vi "Newport ITX-D3N Range Check.vi"(4 "All Out of Range?":bool, 6 "In Range?":bool, 7 "Barometric Pressure":dbl, 8 "Error In":errorcluster, 9 "Humidity":dbl, 10 "Temperature":dbl, 11 "Dewpoint":dbl) -> (0 "Error Out":errorcluster, 1 "Humidity Out":dbl, 2 "Temperature Out":dbl, 3 "Dewpoint Out":dbl, 5 "Barometric Pressure Out":dbl)   [LabVIEW 2020]
uses:
  <vilib>/Analysis/baseanly.llb/Mean (DBL).vi
  <vilib>/Analysis/NI_AALBase.lvlib
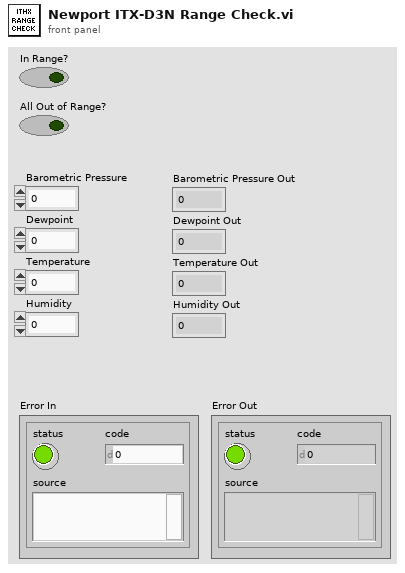
[diagram p1: front panel]
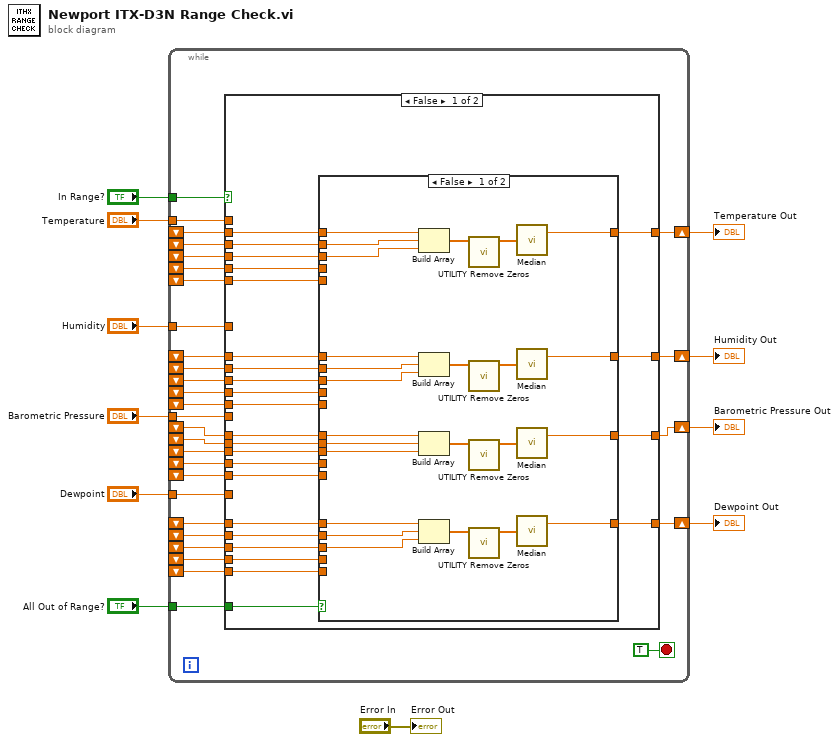
[diagram p0: block diagram]
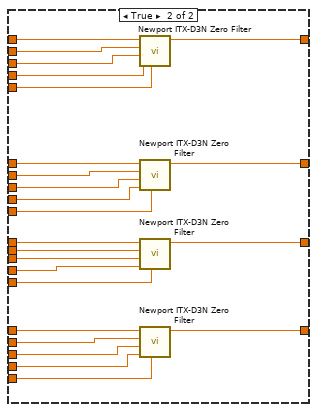
[diagram p2: hidden frame]
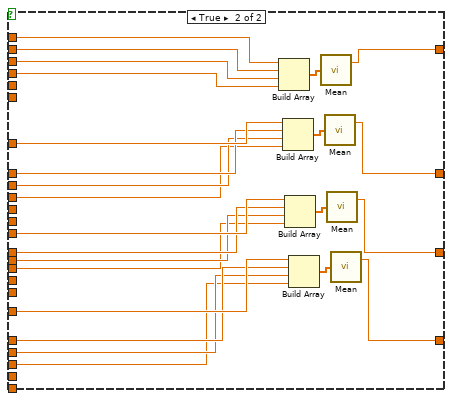
[diagram p3: hidden frame]
diagram:
  n1 = while {
    tunnel: "In Range?" -> [w41]
    shift-right: [w40] -> w9
    shift-left: _ -> [w38]
    tunnel: "Dewpoint" -> [w39]
    tunnel: "Temperature" -> [w37]
    shift-right: [w36] -> w10
    shift-left: _ -> [w33]
    tunnel: "Humidity" -> [w35]
    shift-right: [w34] -> w11
    shift-left: _ -> [w32]
    tunnel: "Barometric Pressure" -> [w31]
    shift-right: [w30] -> w3
    shift-left: _ -> [w29]
    shift-left: _ -> [w22]
    shift-left: _ -> [w21]
    shift-left: _ -> [w28]
    shift-left: _ -> [w27]
    shift-left: _ -> [w26]
    shift-left: _ -> [w25]
    shift-left: _ -> [w24]
    shift-left: _ -> [w23]
    tunnel: "All Out of Range?" -> [w20]
    shift-left: _ -> [w13]
    shift-left: _ -> [w12]
    shift-left: _ -> [w15]
    shift-left: _ -> [w14]
    shift-left: _ -> [w17]
    shift-left: _ -> [w16]
    shift-left: _ -> [w19]
    shift-left: _ -> [w18]
    stop <- TRUE stop-if-true
    n2 = case shown="False" w41 {
      tunnel: w39 -> [_ w130]
      tunnel: [w63 w126] -> w40
      tunnel: w38 -> [w62 w127]
      tunnel: w37 -> [_ w139]
      tunnel: [w56 w123] -> w36
      tunnel: w35 -> [_ w138]
      tunnel: [w52 w124] -> w34
      tunnel: w33 -> [w59 w120]
      tunnel: w32 -> [w55 w135]
      tunnel: [w64 w125] -> w30
      tunnel: w31 -> [_ w134]
      tunnel: w29 -> [w65 w131]
      tunnel: w28 -> [w66 w132]
      tunnel: w27 -> [w67 w133]
      tunnel: w26 -> [w61 w128]
      tunnel: w25 -> [w60 w129]
      tunnel: w24 -> [w58 w121]
      tunnel: w23 -> [w57 w122]
      tunnel: w22 -> [w54 w136]
      tunnel: w21 -> [w53 w137]
      tunnel: w20 -> [w51 _]
      tunnel: w19 -> [w50 _]
      tunnel: w18 -> [w49 _]
      tunnel: w17 -> [w47 _]
      tunnel: w16 -> [w48 _]
      tunnel: w15 -> [w46 _]
      tunnel: w14 -> [w45 _]
      tunnel: w13 -> [w44 _]
      tunnel: w12 -> [w43 _]
      frame False {
        n3 = case shown="False" w51 {
          tunnel: w67 -> [w91 w105]
          tunnel: w66 -> [w90 w104]
          tunnel: w65 -> [w89 w103]
          tunnel: [w88 w94] -> w64
          tunnel: [w87 w95] -> w63
          tunnel: w62 -> [w86 w98]
          tunnel: w61 -> [w85 w99]
          tunnel: w60 -> [w84 w100]
          tunnel: w59 -> [w83 w113]
          tunnel: w58 -> [w82 w112]
          tunnel: w57 -> [w81 w111]
          tunnel: [w80 w92] -> w56
          tunnel: w55 -> [w79 w108]
          tunnel: w54 -> [w78 w109]
          tunnel: w53 -> [w77 w110]
          tunnel: [w76 w93] -> w52
          tunnel: w50 -> [_ w114]
          tunnel: w49 -> [_ w115]
          tunnel: w48 -> [_ w106]
          tunnel: w47 -> [_ w107]
          tunnel: w46 -> [_ w102]
          tunnel: w45 -> [_ w101]
          tunnel: w44 -> [_ w97]
          tunnel: w43 -> [_ w96]
          frame False {
            n4 = Build Array(w81, w82, w83) -> (w75:dbl[])
            n5 = Build Array(w77, w78, w79) -> (w73:dbl[])
            n6 = Build Array(w91, w90, w89) -> (w71:dbl[])
            n7 = Build Array(w84, w85, w86) -> (w69:dbl[])
            n8 = call "UTILITY Remove Zeros.vi"("Array in"=w75) -> ("Array out"=w74:dbl[])  [unwired: 10 in]
            n9 = call "UTILITY Remove Zeros.vi"("Array in"=w73) -> ("Array out"=w72:dbl[])  [unwired: 10 in]
            n10 = call "UTILITY Remove Zeros.vi"("Array in"=w71) -> ("Array out"=w70:dbl[])  [unwired: 10 in]
            n11 = call "UTILITY Remove Zeros.vi"("Array in"=w69) -> ("Array out"=w68:dbl[])  [unwired: 10 in]
            n12 = call <vilib>:"Median.vi"("X"=w74) -> ("median"=w80:dbl)  [unwired: 1 out]
            n13 = call <vilib>:"Median.vi"("X"=w72) -> ("median"=w76:dbl)  [unwired: 1 out]
            n14 = call <vilib>:"Median.vi"("X"=w70) -> ("median"=w88:dbl)  [unwired: 1 out]
            n15 = call <vilib>:"Median.vi"("X"=w68) -> ("median"=w87:dbl)  [unwired: 1 out]
          }
          frame True {
            n16 = call "Newport ITX-D3N Zero Filter.vi"("element 5"=w115, "element 4"=w114, "element 3"=w113, "element 2"=w112, "element"=w111) -> ("median"=w92:dbl)  [unwired: 6 in]
            n17 = call "Newport ITX-D3N Zero Filter.vi"("element 5"=w106, "element 4"=w107, "element 3"=w108, "element 2"=w109, "element"=w110) -> ("median"=w93:dbl)  [unwired: 6 in]
            n18 = call "Newport ITX-D3N Zero Filter.vi"("element 5"=w101, "element 4"=w102, "element 3"=w103, "element 2"=w104, "element"=w105) -> ("median"=w94:dbl)  [unwired: 6 in]
            n19 = call "Newport ITX-D3N Zero Filter.vi"("element 5"=w96, "element 4"=w97, "element 3"=w98, "element 2"=w99, "element"=w100) -> ("median"=w95:dbl)  [unwired: 6 in]
          }
        }
      }
      frame True {
        n20 = Build Array(w139, w122, w121, w120) -> (w117:dbl[])
        n21 = Build Array(w138, w137, w136, w135) -> (w116:dbl[])
        n22 = Build Array(w134, w133, w132, w131) -> (w119:dbl[])
        n23 = Build Array(w130, w129, w128, w127) -> (w118:dbl[])
        n24 = call-poly <vilib>:"Mean.vi"("X"=w117) -> ("mean"=w123:dbl)  [unwired: 1 out]
        n25 = call-poly <vilib>:"Mean.vi"("X"=w116) -> ("mean"=w124:dbl)  [unwired: 1 out]
        n26 = call-poly <vilib>:"Mean.vi"("X"=w119) -> ("mean"=w125:dbl)  [unwired: 1 out]
        n27 = call-poly <vilib>:"Mean.vi"("X"=w118) -> ("mean"=w126:dbl)  [unwired: 1 out]
      }
    }
  }
  "Humidity Out" <- w11
  "Temperature Out" <- w10
  "Dewpoint Out" <- w9
  "Barometric Pressure Out" <- w3
  "Error Out" <- "Error In"
